vi "Ready to insert.vi"(7 "Measurement Names":string[](array[string]), 8 "error in (no error)":errorcluster, 9 "Table description":T2={"ActiveCell"={"Row"=-2, "Column"=-2}, "CellBGColor"=0, "CellFontSize"=20, "CellFontBold"=TRUE, "CellFontColor"=0, "CellJustification"=enum."Center", "CellWidth"=122, "NumberOfRows"=0, "AutosizingRowHeight"=TRUE, "SizeHeight"=105, "Position"={"Left"=0, "Top"=0}, "TableWidth"=0, "RowHeaderHeight"=0, "RowHeaderColor"=0}, 10 "Reference position":T1, 11 "ZenGage v3.0 UI in":refnum<class "ZenGage v3.0 UI.lvclass">) -> (0 "error out":errorcluster, 3 "ZenGage v3.0 UI out":refnum<class "ZenGage v3.0 UI.lvclass">)   [LabVIEW 2015]
uses:
  Type Definitions/General/UI States(UI button enable disable).ctl
  ZenGage v3.0 UI.lvclass
  <vilib>/Utility/miscctls.llb/LVRowAndColumnTypeDef.ctl
  <vilib>/Utility/miscctls.llb/LVPositionTypeDef.ctl
  Type Definitions/Inspection/Table description.ctl
panel:
  in  "config\nimage\nreposition":bool
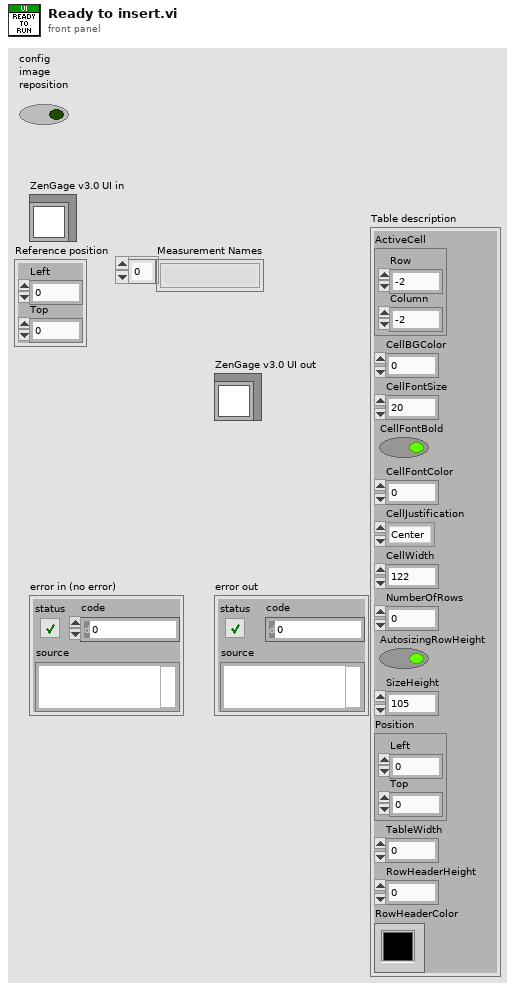
[diagram p1: front panel]
types:
  T1 = typedef "LVPositionTypeDef.ctl" = cluster{"Left":i32, "Top":i32}
  T2 = typedef "ZenGage v3.0 UI.lvclass/Table description.ctl" = cluster{"ActiveCell":T3, "CellBGColor":u32, "CellFontSize":u32, "CellFontBold":bool, "CellFontColor":u32, "CellJustification":enum16{"Left", "Center", "Right"}, "CellWidth":u32, "NumberOfRows":u32, "AutosizingRowHeight":bool, "SizeHeight":u32, "Position":T1, "TableWidth":u32, "RowHeaderHeight":u32, "RowHeaderColor":u32}
  T3 = typedef "LVRowAndColumnTypeDef.ctl" = cluster{"Row":i32, "Column":i32}
  T4 = enum8{"Enabled", "Disabled", "Disabled and Grayed Out"}
  T5 = typedef "ZenGage v3.0 UI.lvclass/UI States(UI button enable disable).ctl" = cluster{"Inspection":cluster{"Inspection States":enum16{"PreSelect", "Back _Inspection", "Analytics", "Ready To Run", "Ready To Insert", "Enable All buttons", "Disable All Buttons", "Settings", "Select", "Stop", "Pause", "Inspect"}}, "Diagnostics":cluster{"Diagnostics States":enum16{"Enable All", "Camera Optics Fail", "Loading Bar", "Camera Optics", "Motor", "Arduino", "POST Done", "POST"}}, "Edit Tolerance":cluster{"Edit Limits":enum16{"Update List"}, "Enable Disable Measurements":enum16{"Back to Edit Tolerance"}, "Page Select":enum16{"Edit Tolerance Limits", "Enable Disable Buttons"}}, "Page Select":enum16{"Edit Tolerance", "Diagnostics", "Inspection"}}
  T6 = enum32{"Analytics", "Blank", "Diagnostics", "Run", "Edit Tolerance Settings"}
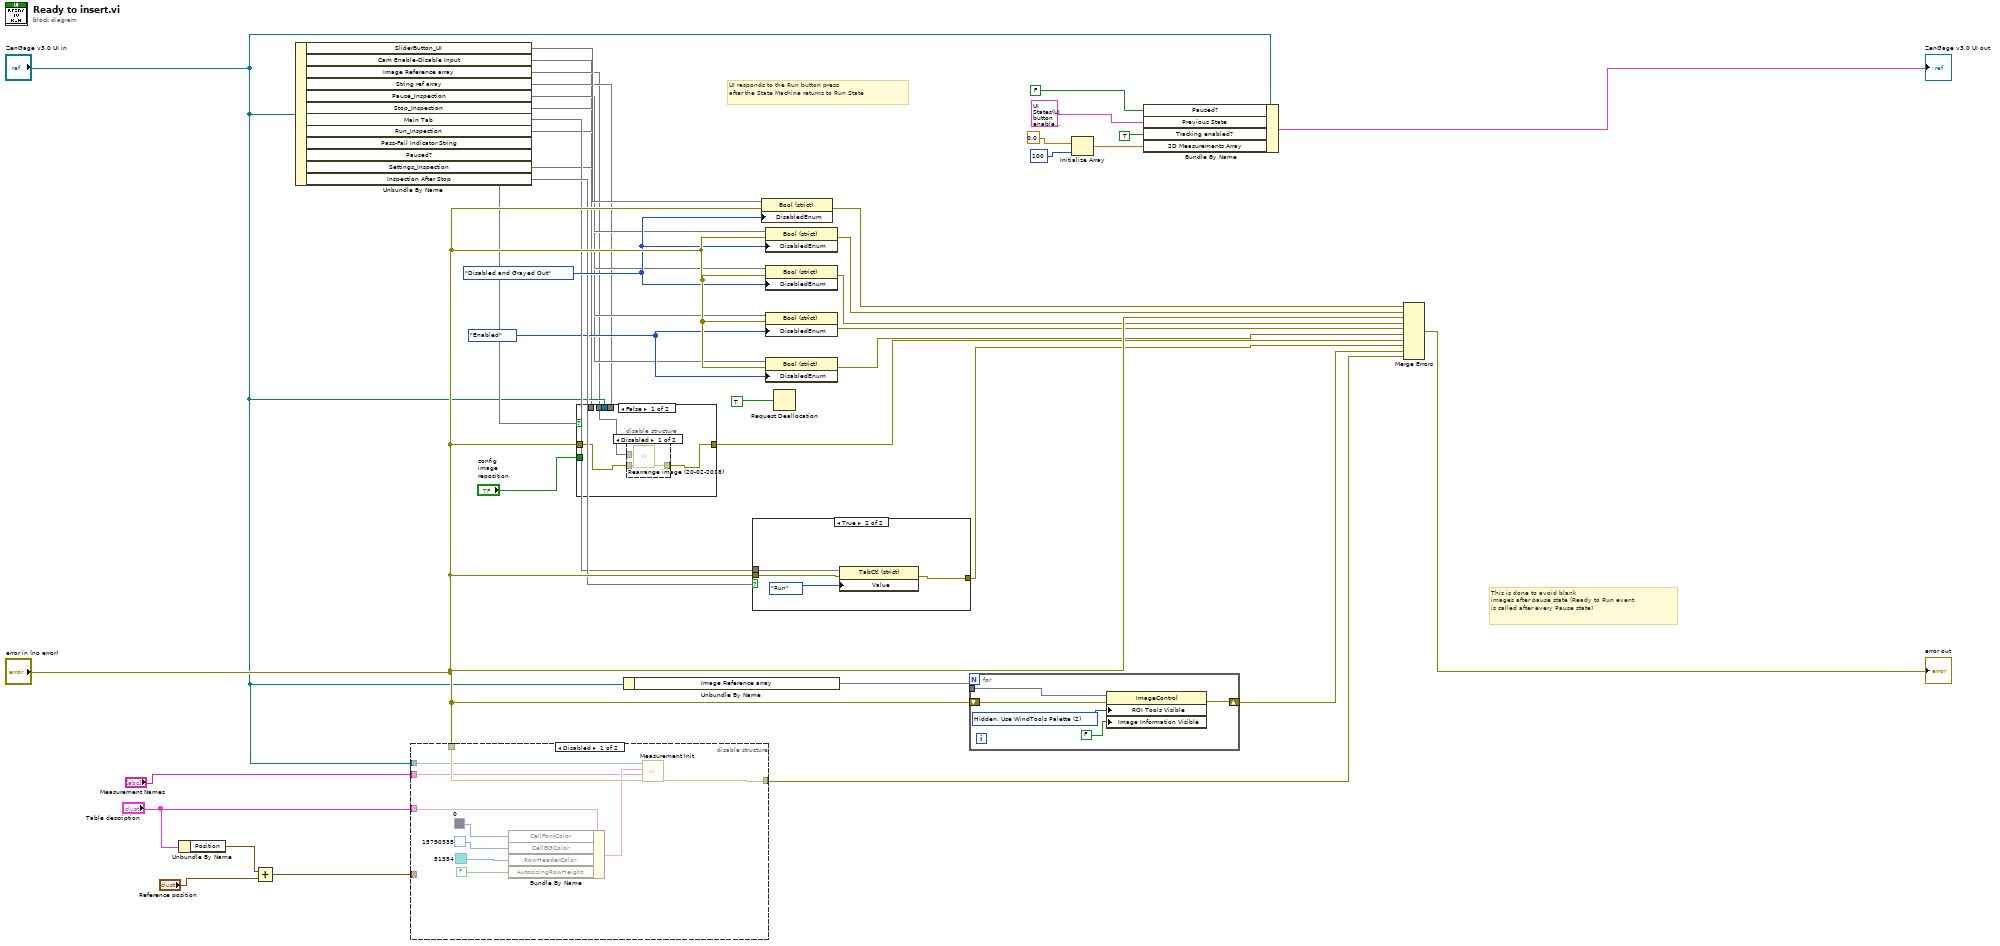
[diagram p0: block diagram]
diagram:
  w36 = T4."Disabled and Grayed Out" ("Disabled")
  w20 = T4."Enabled" ("Disabled")
  # "This is done to avoid blank\nimages after pause state (Ready to Run event\nis called after every Pause state)"
  # "UI responds to the Run button press\nafter the State Machine returns to Run State"
  n1 = Unbundle By Name("Table description") -> ("Position"=w3:T1)
  n2 = Add(x=w3, y="Reference position") -> (x+y=w2:T1)
  n3 = Unbundle By Name("ZenGage v3.0 UI in") -> ("SliderButton_UI"=w37, "Cam Enable-Disable Input"=w12, "Image Reference array"=w13, "String ref array"=w14, "Pause_Inspection"=w19, "Stop_Inspection"=w18, "Main Tab"=w34, "Run_Inspection"=w26, "Paused?"=w33, "Settings_Inspection"=w32, "Inspection After Stop"=w35)  [unwired: 1 out]
  n4 = disable-structure shown="Disabled" {
    disable-tunnel: "error in (no error)" -> [w50 w51]
    disable-tunnel: [w49 w51] -> w31
    disable-tunnel: "ZenGage v3.0 UI in" -> [w48 _]
    disable-tunnel: "Table description" -> [w42 _]
    disable-tunnel: w2 -> [_ _]
    disable-tunnel: "Measurement Names" -> [w41 _]
    frame Disabled {
      n5 = Bundle By Name(cluster=w42, "CellFontColor"=u32 0, "CellBGColor"=u32 15790335, "RowHeaderColor"=u32 51354, "AutosizingRowHeight"=FALSE) -> (w46:T2)
      n6 = call-dynamic "Measurement Init.vi"("error in (no error)"=w50, "Measurement Names"=w41, "Table description"=w46, "ZenGage v3.0 UI in"=w48) -> ("error out"=w49:errorcluster)  [unwired: 6 in, 1 out]
    }
    frame Enabled {
    }
  }
  n7 = case shown="False" w33 {
    tunnel: w12 -> [_ _]
    tunnel: w13 -> [w54 _]
    tunnel: w14 -> [_ _]
    tunnel: [w53 w59] -> w23
    tunnel: "ZenGage v3.0 UI in" -> [_ _]
    tunnel: "error in (no error)" -> [w52 w59]
    tunnel: "config\nimage\nreposition" -> [_ _]
    frame False {
      n8 = disable-structure shown="Disabled" {
        disable-tunnel: w54 -> [w57 _]
        disable-tunnel: [w56 w58] -> w53
        disable-tunnel: w52 -> [w55 w58]
        frame Disabled {
          n9 = call "Rearrange image (20-02-2018).vi"("error in (no error)"=w55, "Image refnum array"=w57) -> ("error out (no error)"=w56:errorcluster)  [unwired: 9 in]
        }
        frame Enabled {
        }
      }
    }
    frame True {
    }
  }
  n10 = Unbundle By Name("ZenGage v3.0 UI in") -> ("Image Reference array"=w28)
  n11 = case shown="True" w35 {
    tunnel: [w60 w64] -> w25
    tunnel: w34 -> [_ w62]
    tunnel: "error in (no error)" -> [w60 w61]
    frame False {
    }
    frame True {
      n12 = property class="TabCtl (strict)"(reference=w62, error in=w61, "Value"=T6."Run") -> (error out=w64:errorcluster)  [unwired: 1 out]
    }
  }
  n13 = property class="Bool (strict)"(reference=w37, error in="error in (no error)", "DisabledEnum"=w36) -> (error out=w39:errorcluster)  [unwired: 1 out]
  n14 = property class="Bool (strict)"(reference=w32, error in="error in (no error)", "DisabledEnum"=w36) -> (error out=w38:errorcluster)  [unwired: 1 out]
  n15 = property class="Bool (strict)"(reference=w26, error in="error in (no error)", "DisabledEnum"=w36) -> (error out=w27:errorcluster)  [unwired: 1 out]
  n16 = property class="Bool (strict)"(reference=w19, error in="error in (no error)", "DisabledEnum"=w20) -> (error out=w21:errorcluster)  [unwired: 1 out]
  n17 = property class="Bool (strict)"(reference=w18, error in="error in (no error)", "DisabledEnum"=w20) -> (error out=w22:errorcluster)  [unwired: 1 out]
  n18 = Request Deallocation(TRUE ("flag")) -> ()
  n19 = for {
    tunnel: w28 -> [w69]
    shift-right: [w66] -> w29
    shift-left: "error in (no error)" -> [w67]
    w68 = u32 2 items=["Visible", "Hidden", "Hidden, Use WindTools Palette"] ("ROI Tools Visible")
    n20 = property class="ImageControl"(reference=w69, error in=w67, "ROI Tools Visible"=w68, "Image Information Visible"=FALSE) -> (error out=w66:errorcluster)  [unwired: 1 out]
  }
  n21 = Initialize Array(0.0 ("element"), 100 ("dimension size")) -> (w17:dbl[])
  n22 = Bundle By Name(cluster="ZenGage v3.0 UI in", "Paused?"=FALSE ("Inspection.Paused?"), "Previous State"=T5 {"Inspection"={"Inspection States"=enum."Ready To Run"}, "Diagnostics"={"Diagnostics States"=enum."Enable All"}, "Edit Tolerance"={"Edit Limits"=enum."Update List", "Enable Disable Measurements"=enum."Back to Edit Tolerance", "Page Select"=enum."Edit Tolerance Limits"}, "Page Select"=enum."Inspection"} ("UI States"), "Tracking enabled?"=TRUE ("Inspection.Tracking enabled?"), "2D Measurements Array"=w17) -> (→"ZenGage v3.0 UI out":cluster{})
  n23 = Merge Errors(w39, w38, "error in (no error)", w27, w21, w22, w23, w25, w29, w31) -> (→"error out":errorcluster)
